vi "Get Phase.vi"(8 "error in (no error)":errorcluster) -> (0 "error out":errorcluster, 3 "function return":dbl)   [LabVIEW 2021, in "vmmso.lvlib"]
doc: "DLL_API double WINAPI GetPhase();"
uses:
  vmmso.lvlib
  vmmso.dll
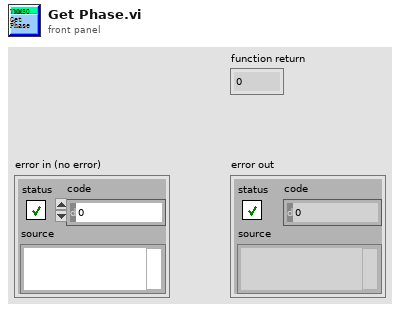
[diagram p1: front panel]
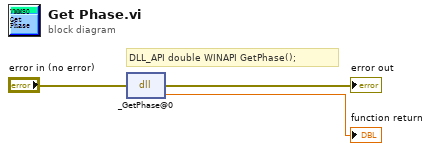
[diagram p0: block diagram]
diagram:
  # "DLL_API double WINAPI GetPhase();"
  n1 = dll-call lib="O:/MSO/library/demo-Labview/vmmso/vmmso.*" fn="_GetPhase@0"(error in="error in (no error)") -> (error out=→"error out":errorcluster, →"function return":dbl)  [unwired: 2 in, 1 out]
